vi "5_VisualAD_HyperParam_Search.vi"() -> ()   [LabVIEW 2020]
uses:
  <vilib>/Ngene/DeepLTK Anomaly Detection Addon/DeepLTK_Anomaly_Detection_Addon/API/Controls/NNPC_Coreset_Params.ctl
  <vilib>/Ngene/DeepLTK Anomaly Detection Addon/DeepLTK_Anomaly_Detection_Addon/API/Controls/NNPC_Setup.ctl
  <vilib>/Ngene/Deep Learning Toolkit/Toolkit/NN_Data/API/NN_Dims(C,H,W).ctl
  <vilib>/Ngene/Deep Learning Toolkit/Toolkit/NN_Network/Controls/NN_Device.ctl
  <vilib>/Ngene/DeepLTK Anomaly Detection Addon/DeepLTK_Anomaly_Detection_Addon/API/Controls/Feature_Scorer_Params.ctl
  <vilib>/Ngene/DeepLTK Anomaly Detection Addon/DeepLTK_Anomaly_Detection_Addon/API/Controls/Gaussian_Blur.ctl
  <vilib>/Ngene/DeepLTK Anomaly Detection Addon/DeepLTK_Anomaly_Detection_Addon/API/Controls/Evaluation_Metrics.ctl
  <vilib>/Ngene/DeepLTK Anomaly Detection Addon/DeepLTK_Anomaly_Detection_Addon/API/Controls/Eval_Results.ctl
  <vilib>/Ngene/DeepLTK Anomaly Detection Addon/DeepLTK_Anomaly_Detection_Addon/API/Controls/MinMax.ctl
  <vilib>/Ngene/DeepLTK Anomaly Detection Addon/DeepLTK_Anomaly_Detection_Addon/API/Controls/NNPC_Random_Projection_CFG.ctl
  <vilib>/Ngene/DeepLTK Anomaly Detection Addon/DeepLTK_Anomaly_Detection_Addon/API/Controls/Dim_Reduction_Method.ctl
  <vilib>/Ngene/DeepLTK Anomaly Detection Addon/DeepLTK_Anomaly_Detection_Addon/API/Controls/NNFE_CFG.ctl
  <vilib>/Ngene/DeepLTK Anomaly Detection Addon/DeepLTK_Anomaly_Detection_Addon/API/Controls/Layer_Selector.ctl
  <vilib>/Ngene/DeepLTK Anomaly Detection Addon/DeepLTK_Anomaly_Detection_Addon/API/Controls/Feature_Layer_Selector.ctl
  <vilib>/Ngene/DeepLTK Anomaly Detection Addon/DeepLTK_Anomaly_Detection_Addon/API/Controls/Interpolation_Selector.ctl
  subVIs/Dataset_Reader/Controls/Read_Options.ctl
  <vilib>/Ngene/DeepLTK Anomaly Detection Addon/DeepLTK_Anomaly_Detection_Addon/API/Controls/NNPC_PreProcessing_Options.ctl
  <vilib>/Ngene/DeepLTK Anomaly Detection Addon/DeepLTK_Anomaly_Detection_Addon/API/Controls/NNPC_DS_Stats.ctl
  <vilib>/Ngene/DeepLTK Anomaly Detection Addon/DeepLTK_Anomaly_Detection_Addon/API/Controls/Image_Stats_RGB.ctl
  subVIs/HyperParam_Investigation/Controls/Model_Info_and_Report.ctl
  subVIs/HyperParam_Investigation/Controls/Feature_Layers_CFG.ctl
  <vilib>/Ngene/DeepLTK Anomaly Detection Addon/DeepLTK_Anomaly_Detection_Addon/API/Controls/Eval_Config.ctl
  <vilib>/Ngene/DeepLTK Anomaly Detection Addon/DeepLTK_Anomaly_Detection_Addon/API/NNPC_Generate_Embedding/NNPC_Generate_Embedding(Dataset).vi
  <vilib>/Ngene/DeepLTK Anomaly Detection Addon/DeepLTK_Anomaly_Detection_Addon/API/NNPC_Predict/NNPC_Predict(Dataset).vi
  <vilib>/Ngene/Deep Learning Toolkit/Toolkit/NN_Data/subVIs/Dataset_Destroy/NN_Dataset_Destroy(In3D_Out3D).vi
  <vilib>/Ngene/DeepLTK Anomaly Detection Addon/DeepLTK_Anomaly_Detection_Addon/API/Controls/NNPC_Save_CFG.ctl
  <vilib>/Ngene/DeepLTK Anomaly Detection Addon/DeepLTK_Anomaly_Detection_Addon/DeepLTK_Anomaly_Detection_Addon.lvlib
  <vilib>/Ngene/Deep Learning Toolkit/Toolkit/Deep_Learning_Toolkit_by_Ngene.lvlib
panel:
  in  "Tab Control":enum32{"Setup", "Results"}(tab)=enum."Results"
  in  "Min_Layers_In_Group":u16=2
  in  "Dataset_Path(Train/Test/GT)":path=path "D:/DNN/_from_Customer/2025_04_11_NIConnect_PCB5/1_Dataset/20_10_Train_2BG_Append_2025_04_21"
  in  "PatchCore_Dest_Folder_Path":path=path "D:/working/HPO_PCB5_Large/RN18"
  in  "Coreset_Size":sgl[](array[numeric])=[15000.0, 20000.0, 25000.0]
  in  "Image Res.":i32[](array[numeric])=[448, 464, 480]
  in  "Proj._Dim.":i32[](array[numeric])=[300]
  in  "Coreset_Params":T1={"CoreSet_Size"=2000.0, "Start_idx"=3}
  in  "NNPC_Setup":T2={"Input_Dims"={"C"=3, "H"=224, "W"=224}, "mBatch"=1, "Device"=enum."GPU", "GPU Id"=0}
  in  "Feature_Scorer_Params":T5={"Nearest_Neighbors"=1, "Calculate Anomaly Map"=FALSE, "Gaussian_Blur"={"Kernel_Size"=33, "Sigma"=4.0}}
  in  "Dim Reduction":T7={"Method"=enum."Rnd_Proj", "Target_Dim"=-1, "Seed"=42}
  in  "NNFE_CFG":T9={"Name"="AD_PCB4", "Layer_Selection_By"=enum."Stride", "Feature_Layers"={"[LayerID, PatchSize]"=[{"Layer_ID"=8, "Patch_Size"=3}, {"Layer_ID"=16, "Patch_Size"=3}]}, "Interpolation_Type"=enum."Bi-Linear"}
  in  "NNFE_Folder_Paths":path[](array[path])=[path "D:/Ngene/Projects_SVN/AD/Models/0_Orig/RN18_1", path "D:/Ngene/Projects_SVN/AD/Models/0_Orig/RN18_2", path "D:/Ngene/Projects_SVN/AD/Models/0_Orig/RN18_3"]
  in  "Patch Sizes":i32[](array[numeric])=[1, 3, 5]
  in  "Layer IDs":i32[](array[numeric])=[8, 16]
  out "Feature_Layers":T11[](array[typedef])=[{"[LayerID, PatchSize]"=[{"Layer_ID"=16, "Patch_Size"=1}]}, {"[LayerID, PatchSize]"=[{"Layer_ID"=16, "Patch_Size"=3}]}, {"[LayerID, PatchSize]"=[{"Layer_ID"=16, "Patch_Size"=5}]}, {"[LayerID, PatchSize]"=[{"Layer_ID"=8, "Patch_Size"=1}]}, {"[LayerID, PatchSize]"=[{"Layer_ID"=8, "Patch_Size"=1}, {"Layer_ID"=16, "Patch_Size"=1}]}, {"[LayerID, PatchSize]"=[{"Layer_ID"=8, "Patch_Size"=1}, {"Layer_ID"=16, "Patch_Size"=3}]}, {"[LayerID, PatchSize]"=[{"Layer_ID"=8, "Patch_Size"=1}, {"Layer_ID"=16, "Patch_Size"=5}]}, {"[LayerID, PatchSize]"=[{"Layer_ID"=8, "Patch_Size"=3}]}, {"[LayerID, PatchSize]"=[{"Layer_ID"=8, "Patch_Size"=3}, {"Layer_ID"=16, "Patch_Size"=1}]}, {"[LayerID, PatchSize]"=[{"Layer_ID"=8, "Patch_Size"=3}, {"Layer_ID"=16, "Patch_Size"=3}]}, {"[LayerID, PatchSize]"=[{"Layer_ID"=8, "Patch_Size"=3}, {"Layer_ID"=16, "Patch_Size"=5}]}, {"[LayerID, PatchSize]"=[{"Layer_ID"=8, "Patch_Size"=5}]}, {"[LayerID, PatchSize]"=[{"Layer_ID"=8, "Patch_Size"=5}, {"Layer_ID"=16, "Patch_Size"=1}]}, {"[LayerID, PatchSize]"=[{"Layer_ID"=8, "Patch_Size"=5}, {"Layer_ID"=16, "Patch_Size"=3}]}, {"[LayerID, PatchSize]"=[{"Layer_ID"=8, "Patch_Size"=5}, {"Layer_ID"=16, "Patch_Size"=5}]}]
  in  "Max_Layers_In_Group":u16=2
  out "Max_Dist":sgl[](graph)
  out "Total Iters":i32=135
  out "Current Iter":i32=1
  out "Coreset Size":i32=3
  out "Proj. Dim.":i32=1
  out "Img Res.":i32=3
  out "Feature_Layers":i32=15
  out "Elapsed Time":dbl=86.03153250000014 format="%<%H:%M:%S>t"
  out "Evaluation_Metrics(Image)":T13={"Scores(Good)"={"X Values"=[2.7319342923164367, 2.7571603751182554, 2.7823864579200746, 2.8076125407218933, 2.8328386235237124, 2.858064706325531, 2.88329078912735, 2.9085168719291685, 2.9337429547309877, 2.9589690375328064, 2.9841951203346255, 3.0094212031364442, 3.034647285938263, 3.0598733687400816, 3.0850994515419004, 3.1103255343437195, 3.1355516171455386, 3.1607776999473574, 3.186003782749176, 3.2112298655509948, 3.2364559483528135, 3.2616820311546326, 3.2869081139564513, 3.3121341967582705, 3.337360279560089, 3.362586362361908, 3.3878124451637266, 3.4130385279655457, 3.4382646107673644, 3.4634906935691836, 3.4887167763710023, 3.513942859172821, 3.5391689419746397, 3.5643950247764584, 3.5896211075782776, 3.6148471903800967, 3.6400732731819154, 3.665299355983734, 3.690525438785553, 3.7157515215873715, 3.7409776043891907, 3.76620368719101, 3.7914297699928285, 3.8166558527946473, 3.841881935596466, 3.8671080183982847, 3.8923341012001034, 3.917560184001923, 3.9427862668037417, 3.9680123496055604, 3.993238432407379, 4.018464515209198, 4.0436905980110165, 4.068916680812835, 4.094142763614655, 4.1193688464164735, 4.144594929218292, 4.169821012020111, 4.1950470948219305, 4.220273177623749, 4.245499260425568, 4.270725343227387, 4.295951426029205, 4.321177508831024, 4.346403591632843, 4.371629674434661, 4.39685575723648, 4.4220818400383, 4.447307922840118, 4.472534005641937, 4.497760088443756, 4.5229861712455754, 4.548212254047394, 4.573438336849213, 4.598664419651032, 4.62389050245285, 4.649116585254669, 4.674342668056488, 4.699568750858306, 4.724794833660126, 4.750020916461945, 4.775246999263763, 4.800473082065583, 4.825699164867402, 4.85092524766922, 4.876151330471039, 4.901377413272858, 4.9266034960746765, 4.951829578876495, 4.977055661678314, 5.002281744480133, 5.027507827281951, 5.05273391008377, 5.07795999288559, 5.103186075687408, 5.128412158489228, 5.153638241291047, 5.178864324092865, 5.204090406894684, 5.229316489696503], "Histogram: h(x)"=[1, 0, 0, 0, 1, 1, 0, 0, 0, 0, 0, 2, 2, 2, 5, 9, 13, 20, 27, 26, 18, 22, 13, 22, 8, 15, 14, 13, 5, 4, 7, 3, 5, 1, 2, 0, 4, 3, 1, 1, 3, 1, 0, 0, 1, 0, 1, 3, 0, 3, 2, 1, 1, 2, 0, 0, 0, 1, 0, 1, 0, 1, 0, 0, 0, 1, 0, 0, 0, 0, 0, 0, 0, 0, 1, 0, 0, 1, 0, 0, 0, 0, 0, 0, 0, 0, 0, 0, 0, 0, 1, 0, 0, 0, 1, 0, 1, 0, 0, 0]}, "Scores(Bad)"={"X Values"=[2.7319342923164367, 2.7571603751182554, 2.7823864579200746, 2.8076125407218933, 2.8328386235237124, 2.858064706325531, 2.88329078912735, 2.9085168719291685, 2.9337429547309877, 2.9589690375328064, 2.9841951203346255, 3.0094212031364442, 3.034647285938263, 3.0598733687400816, 3.0850994515419004, 3.1103255343437195, 3.1355516171455386, 3.1607776999473574, 3.186003782749176, 3.2112298655509948, 3.2364559483528135, 3.2616820311546326, 3.2869081139564513, 3.3121341967582705, 3.337360279560089, 3.362586362361908, 3.3878124451637266, 3.4130385279655457, 3.4382646107673644, 3.4634906935691836, 3.4887167763710023, 3.513942859172821, 3.5391689419746397, 3.5643950247764584, 3.5896211075782776, 3.6148471903800967, 3.6400732731819154, 3.665299355983734, 3.690525438785553, 3.7157515215873715, 3.7409776043891907, 3.76620368719101, 3.7914297699928285, 3.8166558527946473, 3.841881935596466, 3.8671080183982847, 3.8923341012001034, 3.917560184001923, 3.9427862668037417, 3.9680123496055604, 3.993238432407379, 4.018464515209198, 4.0436905980110165, 4.068916680812835, 4.094142763614655, 4.1193688464164735, 4.144594929218292, 4.169821012020111, 4.1950470948219305, 4.220273177623749, 4.245499260425568, 4.270725343227387, 4.295951426029205, 4.321177508831024, 4.346403591632843, 4.371629674434661, 4.39685575723648, 4.4220818400383, 4.447307922840118, 4.472534005641937, 4.497760088443756, 4.5229861712455754, 4.548212254047394, 4.573438336849213, 4.598664419651032, 4.62389050245285, 4.649116585254669, 4.674342668056488, 4.699568750858306, 4.724794833660126, 4.750020916461945, 4.775246999263763, 4.800473082065583, 4.825699164867402, 4.85092524766922, 4.876151330471039, 4.901377413272858, 4.9266034960746765, 4.951829578876495, 4.977055661678314, 5.002281744480133, 5.027507827281951, 5.05273391008377, 5.07795999288559, 5.103186075687408, 5.128412158489228, 5.153638241291047, 5.178864324092865, 5.204090406894684, 5.229316489696503], "Histogram: h(x)"=[0, 0, 0, 0, 0, 0, 0, 0, 0, 0, 0, 0, 0, 0, 0, 0, 0, 0, 0, 0, 0, 0, 0, 0, 0, 0, 0, 0, 1, 0, 1, 0, 2, 1, 3, 1, 2, 6, 5, 4, 2, 0, 6, 6, 8, 6, 6, 8, 5, 7, 6, 6, 4, 6, 4, 6, 6, 8, 7, 2, 4, 6, 4, 5, 2, 3, 7, 1, 6, 1, 1, 1, 1, 1, 4, 1, 3, 5, 1, 0, 1, 1, 2, 1, 1, 1, 0, 0, 0, 0, 0, 0, 0, 0, 0, 0, 0, 0, 0, 1]}, "Eval Stats"={"Scores(Good)"={"Min"=2.7193213, "Max"=5.1506834}, "Scores(Bad)"={"Min"=3.4291687, "Max"=5.2419295}, "# of Samples(Good)"=297, "# of Samples(Bad)"=200, "AUROC"=0.95147306, "F1_Max"=0.90410954, "Thrshld(F1_Max)"=3.54504, "Prec.(F1_Max)"=0.8319328, "Recall(F1_Max)"=0.99, "FPR(F1_Max)"=0.13468014, "FNR(F1_Max)"=0.01}} {"Eval Stats"."Recall(F1_Max)" format="%#.5f"; "Eval Stats"."FPR(F1_Max)" format="%#.5f"; "Eval Stats"."FNR(F1_Max)" format="%#.5f"; "Eval Stats"."Prec.(F1_Max)" format="%#.5f"; "Eval Stats"."F1_Max" format="%#.5f"; "Eval Stats"."AUROC" format="%#.5f"; "Eval Stats"."Scores(Bad)"."Min" format="%#_5g"; "Eval Stats"."Scores(Good)"."Min" format="%#_5g"; "Eval Stats"."Thrshld(F1_Max)" format="%#_5f"}
  out "Evaluation_Metrics(Pixel)":T13 {"Eval Stats"."Recall(F1_Max)" format="%#.5f"; "Eval Stats"."FPR(F1_Max)" format="%#.5f"; "Eval Stats"."FNR(F1_Max)" format="%#.5f"; "Eval Stats"."Prec.(F1_Max)" format="%#.5f"; "Eval Stats"."F1_Max" format="%#.5f"; "Eval Stats"."AUROC" format="%#.5f"; "Eval Stats"."Scores(Bad)"."Min" format="%#_5g"; "Eval Stats"."Scores(Good)"."Min" format="%#_5g"; "Eval Stats"."Thrshld(F1_Max)" format="%#_5f"}
  out "Coreset Size":i32=1
  out "Coreset Size":sgl=20000.0
  out "Proj. Dim.":i32=300
  out "Img. Res.":i32=448
  out "Proj. Dim.":i32
  out "Img Res.":i32
  out "dT_Eval":dbl=0.21638530000018363 format="%#_4p"
  out "dT_Inference":dbl=0.004835436016095979 format="%#_4p"
  out "dT_Coreset":dbl=52.57081759999983 format="%#_4p"
  out "dT_Embed":dbl=4.344940299999962 format="%#_3p"
  out "dT_Init":dbl=0.7978293999999551 format="%#_3p"
  out "dT_DS_Read(Test)":dbl=6.224915199999941 format="%#_3p"
  out "dT_DS_Read(Train)":dbl=16.388801800000238 format="%#_3p"
  out "DS Size(Test)":i32=497
  out "DS Size(Train)":i32=1036
  out "Feature_Layers":i32
  out "error out":errorcluster
  out "dT_DS_Read(Train)":dbl=48.993010699999985
  out "dT_DS_Read(Test)":dbl=18.836170100000004
  out "dT_Init":dbl=2.419111600000008
  out "dT_Predict":dbl=8.196476700000034
  out "dT_Coreset":dbl=154.10587869999995
  out "dT_Embed":dbl=13.308446900000035
  out "dT_Eval":dbl=0.7761126999999419
  out "Feature Extractor":string="rn18_2"
  out "dT_Predict":dbl=2.4032116999997015
  out "[LayerID, PatchSize]":cluster{"Layer_ID":i32, "Patch_Size":i32}[](array[cluster])=[{"Layer_ID"=16, "Patch_Size"=1}]
  in  "Stop":bool
  out "NNFE":i32=1
  out "NNFE":i32=3
  # "Total Iterations"
  # "Current Iteration"
  # "Current Settings"
  # "Total Times"
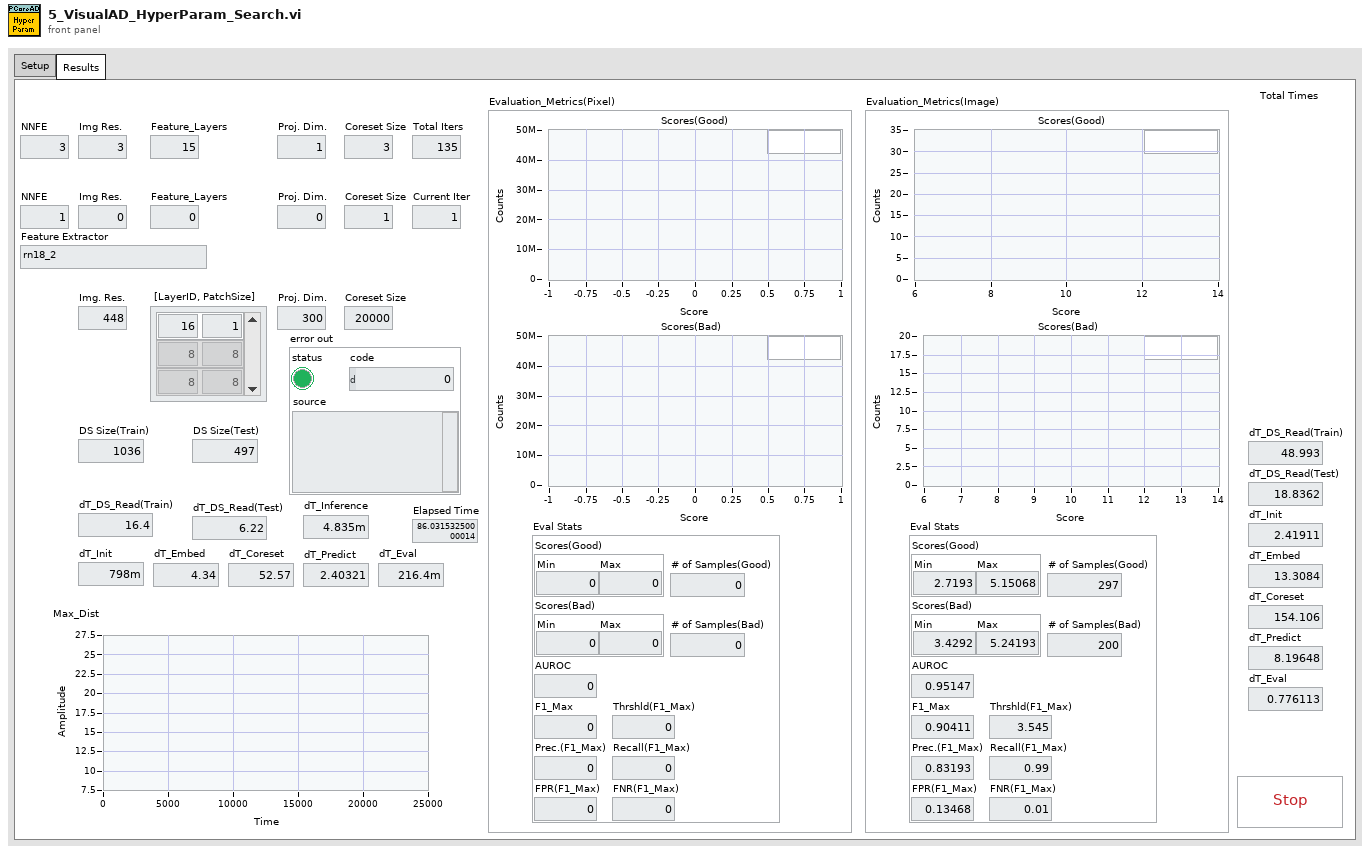
[diagram p1: front panel]
types:
  T1 = typedef "DeepLTK_Anomaly_Detection_Addon.lvlib/NNPC_Coreset_Params.ctl" = cluster{"CoreSet_Size":sgl, "Start_idx":i32}
  T2 = typedef "DeepLTK_Anomaly_Detection_Addon.lvlib/NNPC_Setup.ctl" = cluster{"Input_Dims":T3, "mBatch":i32, "Device":T4, "GPU Id":i32}
  T3 = typedef "Deep_Learning_Toolkit_by_Ngene.lvlib/NN_Dims(C,H,W).ctl" = cluster{"C":i32, "H":i32, "W":i32}
  T4 = typedef "Deep_Learning_Toolkit_by_Ngene.lvlib/NN_Device.ctl" = enum16{"CPU", "GPU"}
  T5 = typedef "DeepLTK_Anomaly_Detection_Addon.lvlib/Feature_Scorer_Params.ctl" = cluster{"Nearest_Neighbors":i32, "Calculate Anomaly Map":bool, "Gaussian_Blur":T6}
  T6 = typedef "DeepLTK_Anomaly_Detection_Addon.lvlib/Gaussian_Blur.ctl" = cluster{"Kernel_Size":i32, "Sigma":sgl}
  T7 = typedef "DeepLTK_Anomaly_Detection_Addon.lvlib/NNPC_Random_Projection_CFG.ctl" = cluster{"Method":T8, "Target_Dim":i32, "Seed":i32}
  T8 = typedef "DeepLTK_Anomaly_Detection_Addon.lvlib/Dim_Reduction_Method.ctl" = enum16{"None", "Rnd_Proj", "PCA"}
  T9 = typedef "DeepLTK_Anomaly_Detection_Addon.lvlib/NNFE_CFG.ctl" = cluster{"Name":string, "Layer_Selection_By":T10, "Feature_Layers":T11, "Interpolation_Type":T12}
  T10 = typedef "DeepLTK_Anomaly_Detection_Addon.lvlib/Layer_Selector.ctl" = enum16{"Stride", "Layer_Idx"}
  T11 = typedef "DeepLTK_Anomaly_Detection_Addon.lvlib/Feature_Layer_Selector.ctl" = cluster{"[LayerID, PatchSize]":cluster{"Layer_ID":i32, "Patch_Size":i32}[]}
  T12 = typedef "DeepLTK_Anomaly_Detection_Addon.lvlib/Interpolation_Selector.ctl" = enum16{"Nearest", "Bi-Linear"}
  T13 = typedef "DeepLTK_Anomaly_Detection_Addon.lvlib/Evaluation_Metrics.ctl" = cluster{"Scores(Good)":cluster{"X Values":dbl[], "Histogram: h(x)":i32[]}, "Scores(Bad)":cluster{"X Values":dbl[], "Histogram: h(x)":i32[]}, "Eval Stats":T14}
  T14 = typedef "DeepLTK_Anomaly_Detection_Addon.lvlib/Eval_Results.ctl" = cluster{"Scores(Good)":T15, "Scores(Bad)":T15, "# of Samples(Good)":i32, "# of Samples(Bad)":i32, "AUROC":sgl, "F1_Max":sgl, "Thrshld(F1_Max)":sgl, "Prec.(F1_Max)":sgl, "Recall(F1_Max)":sgl, "FPR(F1_Max)":sgl, "FNR(F1_Max)":sgl}
  T15 = typedef "DeepLTK_Anomaly_Detection_Addon.lvlib/MinMax.ctl" = cluster{"Min":sgl, "Max":sgl}
  T16 = typedef "DeepLTK_Anomaly_Detection_Addon.lvlib/NN_Paths.ctl" = cluster{"CFG":path, "BIN":path}
  T17 = typedef "DeepLTK_Anomaly_Detection_Addon.lvlib/NNPC_PreProcessing_Options.ctl" = cluster{"DS_Name":string, "Input_Dims":T3, "Center Crop Size":i32, "Interpolation Type":u32, "Multi-Stage_DownSample?":bool, "Dataset_Stats":T18}
  T18 = typedef "DeepLTK_Anomaly_Detection_Addon.lvlib/NNPC_DS_Stats.ctl" = cluster{"means":T19, "stds":T19}
  T19 = typedef "DeepLTK_Anomaly_Detection_Addon.lvlib/Image_Stats_RGB.ctl" = cluster{"R":sgl, "G":sgl, "B":sgl}
  T20 = typedef "Read_Options.ctl" = cluster{"Read Bads?":bool, "Read GTs?":bool, "Update. DS Stats?":bool}
  T21 = typedef "DeepLTK_Anomaly_Detection_Addon.lvlib/Eval_Config.ctl" = cluster{"Extract_Good_Pixels_from_Bad":bool, "# bins":i32}
  T22 = typedef "Model_Info_and_Report.ctl" = cluster{"Name":string, "Feature Extractor":string, "Input3D_Custom_Dims":T3, "Coreset Size":i32, "J-L Proj. Dim.":i32, "Train_Time":dbl, "Inf_Time":dbl, "Feature_Layers":T23, "Eval Stats(Image)":T14, "Eval Stats(Pixel)":T14}
  T23 = typedef "Feature_Layers_CFG.ctl" = cluster{"Layer_ID":i32, "Patch_Size":i32}[]
  T24 = typedef "DeepLTK_Anomaly_Detection_Addon.lvlib/NNPC_Save_CFG.ctl" = cluster{"Add_TimeStamp_SubFolder":bool, "Append_TimeStamp_to_FileNames":bool}
  T25 = typedef "Deep_Learning_Toolkit_by_Ngene.lvlib/NN_DataSet(In3D_Out3D).ctl" = cluster{"Dataset_Size":i32, "Dims_In":T3, "Labels":string[], "File Paths":path[], "Outputs Ref.":T26, "Inputs Ref.":variant, "Dims_Out":T3}
  T26 = typedef "Deep_Learning_Toolkit_by_Ngene.lvlib/NN_Data_ref(4D_SGL).ctl" = refnum<data-value>
  T27 = typedef "DeepLTK_Anomaly_Detection_Addon.lvlib/NNPC_Instance.ctl" = cluster{"NN":T28, "MemBank_Data":T43, "Name":string}
  T28 = typedef "Deep_Learning_Toolkit_by_Ngene.lvlib/NN.ctl" = cluster{"Name":string, "No of Layers":i32, "mBatch":i32, "Layers":T29[], "Dimty":T30, "Dims_In":T3, "Dims_Out":T3, "Working_Dir":path, "Train?":bool, "Train_Params":T31, "LR_Update_Policy":T34, "Session Data":T36, "Ground_truth":T37, "NNg_hdls":T38, "NN_Device":T4, "GPU Id":i32, "Labels":string[], "Receptive Field":T39[], "Loss_Type":T40, "Loss_Cfg_Prms":variant, "NNG_WS":T41}
  T29 = typedef "Deep_Learning_Toolkit_by_Ngene.lvlib/NN_Layer_ref.ctl" = refnum<data-value>
  T30 = typedef "Deep_Learning_Toolkit_by_Ngene.lvlib/NN_In_Out_Dim-ty.ctl" = enum8{"In1D_Out1D", "In3D_Out1D", "In3D_Out3D", "In3D_OutBBox"}
  T31 = typedef "Deep_Learning_Toolkit_by_Ngene.lvlib/NN_Train_Params.ctl" = cluster{"Optimizer":T32, "Beta_1":sgl, "Beta_2":sgl, "Weight Decay(L1)":sgl, "Weight Decay(L2)":sgl, "Data_Sampling":T33}
  T32 = typedef "Deep_Learning_Toolkit_by_Ngene.lvlib/NN_Train_Optimizer.ctl" = enum16{"SGD", "Adam", "Adagrad", "Adadelta", "RMSProp", "Nesterov"}
  T33 = typedef "Deep_Learning_Toolkit_by_Ngene.lvlib/NN_Train_Data_Sampling.ctl" = enum16{"Random", "Sequential"}
  T34 = typedef "Deep_Learning_Toolkit_by_Ngene.lvlib/NN_LR_Policy_Cfg.ctl" = cluster{"Policy_Type":T35, "LR0":dbl, "k":sgl, "WarmUp_Policy":enum16{"Step", "Ramp"}, "WarmUp_Iter":i32, "WarmUp_Ratio":sgl}
  T35 = typedef "Deep_Learning_Toolkit_by_Ngene.lvlib/NN_LR_Policy_Type.ctl" = enum16{"Manual", "Step", "Exp", "1/t"}
  T36 = typedef "Deep_Learning_Toolkit_by_Ngene.lvlib/NN_Train_Session_Data.ctl" = cluster{"Epochs":sgl, "Tot_Iter":i32, "LR":sgl, "LR_iter":i32}
  T37 = typedef "Deep_Learning_Toolkit_by_Ngene.lvlib/NN_Ground_truth.ctl" = cluster{"Y":variant}
  T38 = typedef "Deep_Learning_Toolkit_by_Ngene.lvlib/nng_cuda_handles.ctl" = cluster{"cudnn":u64, "cublas":u64, "stream":u64, "curand":u64}
  T39 = typedef "Deep_Learning_Toolkit_by_Ngene.lvlib/NN_Dims(V,H).ctl" = cluster{"V":i32, "H":i32}
  T40 = typedef "Deep_Learning_Toolkit_by_Ngene.lvlib/NN_Loss_Type.ctl" = enum16{"None", "MSE", "CrossEntropy", "YOLO_v2", "YOLO_v4"}
  T41 = typedef "Deep_Learning_Toolkit_by_Ngene.lvlib/NNG_WS.ctl" = cluster{"NNG_WS_Mem":T42, "Max_WS_Size":i64}
  T42 = typedef "Deep_Learning_Toolkit_by_Ngene.lvlib/NNg_WS_Mem_DVR.ctl" = refnum<data-value>
  T43 = typedef "DeepLTK_Anomaly_Detection_Addon.lvlib/MemBank_and_Norm_Variants.ctl" = cluster{"MemBank":variant, "MemBank Norm":variant}
  T44 = typedef "DeepLTK_Anomaly_Detection_Addon.lvlib/Evaluation_Metrics(Pixel_Image).ctl" = cluster{"Evaluation_Metrics(Pixel)":T13, "Evaluation_Metrics(Image)":T13}
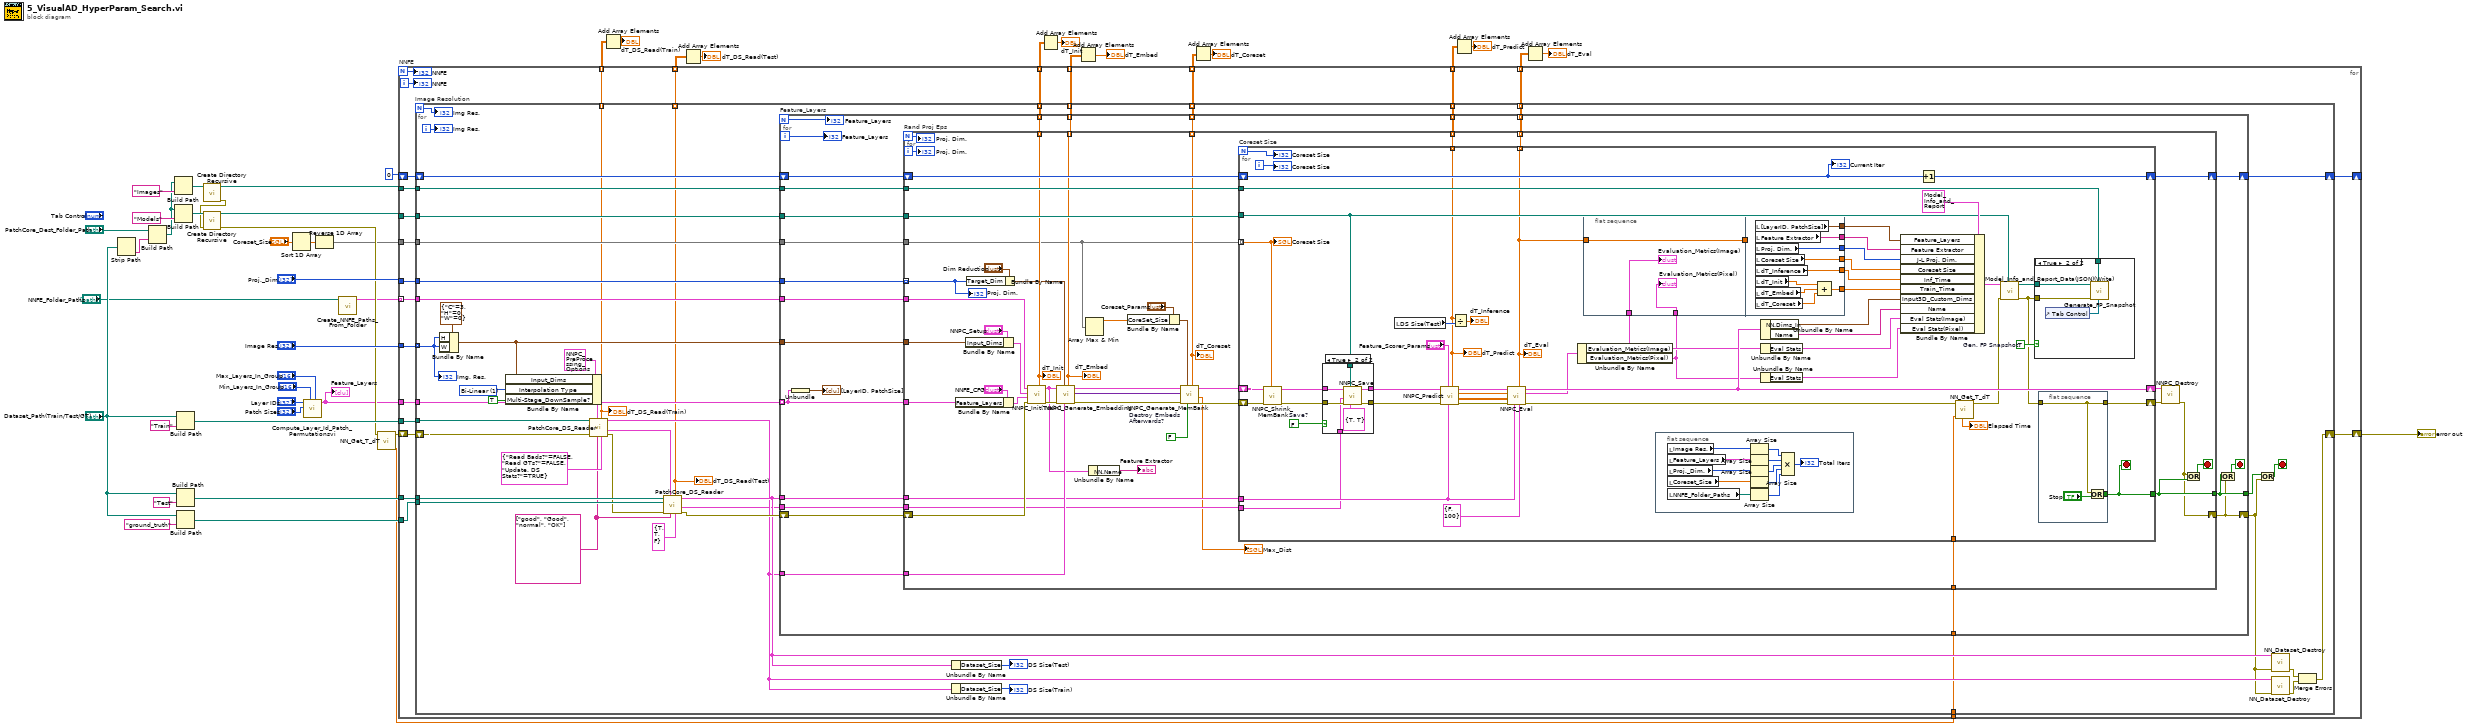
[diagram p0: block diagram]
diagram:
  n1 = Strip Path(path="Dataset_Path(Train/Test/GT)") -> (name=w43:string)  [unwired: 1 out]
  n2 = Build Path(base path="PatchCore_Dest_Folder_Path", name or relative path=w43) -> (appended path=w33:path)
  n3 = Build Path(base path=w33, name or relative path="Images" ("String")) -> (appended path=w37:path)
  n4 = Build Path(base path=w33, name or relative path="Models" ("String")) -> (appended path=w36:path)
  n5 = Build Path(base path="Dataset_Path(Train/Test/GT)", name or relative path="Train" ("String")) -> (appended path=w38:path)
  n6 = Build Path(base path="Dataset_Path(Train/Test/GT)", name or relative path="Test" ("String")) -> (appended path=w39:path)
  n7 = Build Path(base path="Dataset_Path(Train/Test/GT)", name or relative path="ground_truth" ("String")) -> (appended path=w44:path)
  n8 = call <vilib>:"Create Directory Recursive.vi"("directory"=w37) -> ("error out"=w29:errorcluster, "directory copy"=w31:path)  [unwired: 4 in, 1 out]
  n9 = call <vilib>:"Create Directory Recursive.vi"("error in (no error)"=w29, "directory"=w36) -> ("error out"=w28:errorcluster, "directory copy"=w32:path)  [unwired: 3 in, 1 out]
  n10 = Sort 1D Array(array="Coreset_Size") -> (sorted array=w15:sgl[])
  n11 = call "Compute_Layer_Id_Patch_Permutationsvi.vi"("Max Layers"="Max_Layers_In_Group", "Min Layers"="Min_Layers_In_Group", "Patch Sizes"="Patch Sizes", "Layer IDs"="Layer IDs") -> ("LayerID,PatchSize Permutations"=w3:T11[])  [unwired: 7 in]
  "Feature_Layers" <- w3
  n12 = Reverse 1D Array(array=w15) -> (reversed array=w14:sgl[])
  n13 = call "Create_NNFE_Paths_From_Folder.vi"("NNFE_Folder_Paths"="NNFE_Folder_Paths") -> ("NNFE_File_Paths"=w10:T16[])  [unwired: 10 in]
  n14 = call <vilib>:"NN_Get_T_dT.vi"("error in (no error)"=w28) -> ("T_out"=w30:dbl, "error out"=w11:errorcluster)  [unwired: 6 in, 1 out]
  n15 = for "NNFE" {
    N -> [w50]
    tunnel: "Image Res." -> [w72]
    tunnel: w44 -> [w71]
    tunnel: "Proj._Dim." -> [w70]
    tunnel: w39 -> [w69]
    tunnel: w38 -> [w68]
    tunnel: w32 -> [w67]
    tunnel: w31 -> [w66]
    tunnel: w30 -> [w65]
    tunnel: w3 -> [w64]
    tunnel: [w62] -> w26 mode=indexing
    tunnel: [w61] -> w25 mode=indexing
    tunnel: [w60] -> w24 mode=indexing
    tunnel: [w59] -> w23 mode=indexing
    tunnel: [w58] -> w22 mode=indexing
    tunnel: w14 -> [w57]
    shift-right: [w56] -> w12
    shift-left: w11 -> [w55]
    tunnel: w10 -> [w54] mode=indexing
    shift-right: [w53] -> _
    shift-left: 0 ("Img. Res. 2") -> [w63]
    tunnel: [w52] -> w8 mode=indexing
    tunnel: [w51] -> w6 mode=indexing
    i -> [w49]
    n16 = for "Image Resolution" {
      N -> [w90]
      tunnel: w71 -> [w112]
      tunnel: w68 -> [w113]
      tunnel: w72 -> [w115] mode=indexing
      tunnel: w70 -> [w117]
      tunnel: w57 -> [w116]
      tunnel: w69 -> [w111]
      shift-right: [w99] -> w56
      shift-left: w55 -> [w114]
      tunnel: w67 -> [w102]
      tunnel: w66 -> [w101]
      tunnel: w65 -> [w100]
      tunnel: w64 -> [w91]
      shift-right: [w87] -> w53
      shift-left: w63 -> [w88]
      tunnel: [w75] -> w62 mode=indexing
      tunnel: [w74] -> w61 mode=indexing
      tunnel: [w86] -> w60 mode=indexing
      tunnel: [w85] -> w52 mode=indexing
      tunnel: [w84] -> w59 mode=indexing
      tunnel: [w83] -> w58 mode=indexing
      tunnel: [w82] -> w51 mode=indexing
      tunnel: w54 -> [w76]
      i -> [w118]
      stop <- w81 stop-if-true
      w97 = u32 1 items=["Zero Order", "Bi-Linear", "Quadratic", "Cubic Spline"] ("Interpolation Type")
      w77 = string[] ["good", "Good", "normal", "OK"] ("Good Folder Name")
      n17 = Bundle By Name(cluster=T3 {"C"=3, "H"=0, "W"=0} ("Input_Dims"), "H"=w115, "W"=w115) -> (w92:T3)
      n18 = Bundle By Name(cluster=T17 {"DS_Name"="", "Input_Dims"={"C"=4, "H"=224, "W"=224}, "Center Crop Size"=-1, "Interpolation Type"=1, "Multi-Stage_DownSample?"=FALSE, "Dataset_Stats"={"means"={"R"=0.5385, "G"=0.5348, "B"=0.551}, "stds"={"R"=0.3673, "G"=0.3673, "B"=0.3505}}} ("PreProcessing_Options"), "Input_Dims"=w92, "Interpolation Type"=w97, "Multi-Stage_DownSample?"=TRUE) -> (w79:T17)
      n19 = call "PatchCore_DS_Reader.vi"("Read Options"=T20 {"Read Bads?"=FALSE, "Read GTs?"=FALSE, "Update. DS Stats?"=TRUE}, "Good Unique Labels"=w77, "PreProc_Options_in"=w79, "error in (no error)"=w114, "Folder Path"=w113) -> ("error out"=w110:errorcluster, "PreProc_Options_out"=w78:T17, "Dataset"=w104:T25, "dT_DS_Reader"=w75:dbl)  [unwired: 3 in]
      "dT_DS_Read(Train)" <- w75
      n20 = call "PatchCore_DS_Reader.vi"("Read Options"=T20 {"Read Bads?"=TRUE, "Read GTs?"=TRUE, "Update. DS Stats?"=FALSE}, "Good Unique Labels"=w77, "PreProc_Options_in"=w78, "error in (no error)"=w110, "GT Folder Path"=w112, "Folder Path"=w111) -> ("error out"=w108:errorcluster, "PreProc_Options_out"=w94:T17, "Dataset"=w105:T25, "dT_DS_Reader"=w74:dbl)  [unwired: 2 in]
      "dT_DS_Read(Test)" <- w74
      n21 = for "Feature_Layers" {
        N -> [w131]
        tunnel: w117 -> [w143]
        tunnel: w116 -> [w142]
        tunnel: w105 -> [w140]
        tunnel: w104 -> [w139]
        tunnel: w102 -> [w138]
        tunnel: w101 -> [w137]
        tunnel: w100 -> [w136]
        tunnel: w94 -> [w135]
        shift-right: [w121] -> w80
        shift-left: w108 -> [w141]
        tunnel: w92 -> [w133]
        tunnel: w91 -> [w132] mode=indexing
        tunnel: [w130] -> w89
        shift-right: [w129] -> w87
        shift-left: w88 -> [w128]
        tunnel: [w127] -> w86 mode=indexing
        tunnel: [w126] -> w85 mode=indexing
        tunnel: [w125] -> w84 mode=indexing
        tunnel: [w124] -> w83 mode=indexing
        tunnel: [w123] -> w82 mode=indexing
        tunnel: w76 -> [w119]
        i -> [w134]
        stop <- w122 stop-if-true
        n22 = Unbundle(w132) -> ("[LayerID, PatchSize]"=→"[LayerID, PatchSize]":cluster{"Layer_ID":i32, "Patch_Size":i32}[])
        n23 = for "Rand Proj Eps" {
          N -> [w171]
          tunnel: w138 -> [w188]
          tunnel: w139 -> [w183]
          tunnel: w143 -> [w178] mode=indexing
          tunnel: w142 -> [w146]
          shift-right: [w162] -> w121
          shift-left: w141 -> [w187]
          tunnel: w140 -> [w181]
          tunnel: w137 -> [w180]
          tunnel: w136 -> [w179]
          tunnel: w135 -> [w177]
          tunnel: w133 -> [w173]
          tunnel: w132 -> [w172]
          tunnel: [w170] -> w130
          shift-right: [w168] -> w129
          shift-left: w128 -> [w169]
          tunnel: [w167] -> w127 mode=indexing
          tunnel: [w166] -> w126 mode=indexing
          tunnel: [w150] -> w125 mode=indexing
          tunnel: [w165] -> w124 mode=indexing
          tunnel: [w164] -> w123 mode=indexing
          tunnel: w119 -> [w145]
          i -> [w186]
          stop <- w163 stop-if-true
          w154 = FALSE  # Destroy Embeds Afterwards?
          n24 = Bundle By Name(cluster="NNFE_CFG", "Feature_Layers"=w172) -> (w161:T9)
          n25 = Bundle By Name(cluster="NNPC_Setup", "Input_Dims"=w173) -> (w160:T2)
          n26 = Bundle By Name(cluster="Dim Reduction", "Target_Dim"=w178) -> (w159:T7)
          n27 = call <vilib>:"NNPC_Init(Train).vi"("error in"=w187, "NNFE_CFG"=w161, "NNPC_Setup"=w160, "NNFE_Paths"=w145) -> ("error out"=w184:errorcluster, "NNPC_out"=w158:T27, "dT_Init_Train"=w167:dbl)  [unwired: 5 in]
          "dT_Init" <- w167
          n28 = call-poly <vilib>:"NNPC_Generate_Embedding.vi"("Dataset"=w183, "Dim_Reduction"=w159, "error in"=w184, "NNPC_in"=w158) -> ("error out"=w153:errorcluster, "Feature_Embeddings"=w152:variant, "NNPC_out"=w151:T27, "dT_Embed"=w166:dbl)  [unwired: 3 in, 1 out]
          "dT_Embed" <- w166
          n29 = Array Max & Min(array=w146) -> (max value=w149:sgl)  [unwired: 3 out]
          n30 = Unbundle By Name(w158) -> ("NN.Name"=→"Feature Extractor":string)
          n31 = Bundle By Name(cluster="Coreset_Params", "CoreSet_Size"=w149) -> (w156:T1)
          n32 = call <vilib>:"NNPC_Generate_MemBank.vi"("Destroy Embeds Afterwards?"=w154, "Coreset_Params"=w156, "error in (no error)"=w153, "Feature_Embeddings"=w152, "NNPC_in"=w151) -> ("error out"=w148:errorcluster, "Max_Distances"=→"Max_Dist":sgl[], "NNPC_out"=w147:T27, "dT_Coreset"=w150:dbl)  [unwired: 3 in]
          "dT_Coreset" <- w150
          n33 = for "Coreset Size" {
            N -> [w210]
            tunnel: w188 -> [w218]
            shift-right: [w217] -> w185
            shift-left: w147 -> [w196]
            shift-right: [w189] -> w182
            shift-left: w148 -> [w194]
            tunnel: w181 -> [w231]
            tunnel: w180 -> [w220]
            tunnel: w179 -> [w216]
            tunnel: w177 -> [w211]
            tunnel: [w208] -> w170
            shift-right: [w204] -> w168
            shift-left: w169 -> [w205]
            tunnel: [w203] -> w165 mode=indexing
            tunnel: [w202] -> w164 mode=indexing
            tunnel: w146 -> [w192] mode=indexing
            i -> [w240]
            stop <- w208 stop-if-true
            w221 = TRUE  # Gen. FP Snapshot?
            w229 = FALSE  # Save?
            n34 = call <vilib>:"NNPC_Shrink_MemBank.vi"("Coreset_Size"=w192, "error in (no error)"=w194, "NNPC_in"=w196) -> ("error out"=w193:errorcluster, "NNPC_out"=w195:T27)  [unwired: 7 in]
            n35 = case shown="True" w229 {
              tunnel: w218 -> [_ w279]
              tunnel: w193 -> [w271 w278]
              tunnel: w195 -> [w272 w277]
              tunnel: [w271 w275] -> w232
              tunnel: [w272 w274] -> w230
              tunnel: w211 -> [_ w273]
              frame False {
              }
              frame True {
                n36 = call <vilib>:"NNPC_Save.vi"("Save_Config"=T24 {"Add_TimeStamp_SubFolder"=TRUE, "Append_TimeStamp_to_FileNames"=TRUE} ("Save Config"), "Dst_Folder"=w279, "error in (no error)"=w278, "PreProc_Options_in"=w273, "NNPC_in"=w277) -> ("error out"=w275:errorcluster, "NNPC_out"=w274:T27)  [unwired: 4 in, 1 out]
              }
            }
            n37 = local read "DS Size(Test)"() -> (w227:i32)
            n38 = call-poly <vilib>:"NNPC_Predict.vi"("Dataset"=w231, "Feature_Scorer_Params"="Feature_Scorer_Params", "error in (no error)"=w232, "NNPC_in"=w230) -> ("error out"=w235:errorcluster, "Anomaly_Maps"=w234:sgl[][][], "Pred_Scores"=w236:sgl[], "NNPC_out"=w237:T27, "dT_Predict"=w203:dbl)  [unwired: 3 in]
            "dT_Predict" <- w203
            n39 = Divide(x=w203, y=w227) -> (x/y=→"dT_Inference":dbl)
            n40 = call <vilib>:"NNPC_Eval.vi"("Eval_Config"=T21 {"Extract_Good_Pixels_from_Bad"=FALSE, "# bins"=100} ("Eval Config"), "Dataset"=w231, "error in (no error)"=w235, "Anomaly_Maps"=w234, "Pred_Scores"=w236, "NNPC_in"=w237) -> ("error out"=w209:errorcluster, "Evaluation_Metrics"=w206:T44, "NNPC_out"=w217:T27, "dT_Eval"=w202:dbl)  [unwired: 2 in]
            "dT_Eval" <- w202
            n41 = Unbundle By Name(w206) -> ("Evaluation_Metrics(Image)"=w199:T13, "Evaluation_Metrics(Pixel)"=w198:T13)
            n42 = flat-sequence {
              tunnel: w202 -> [w257]
              tunnel: [w257] -> w207
              tunnel: w198 -> [w256]
              tunnel: w199 -> [w255]
              tunnel: [w263] -> w226
              tunnel: [w262] -> w214
              tunnel: [w261] -> w213
              tunnel: [w260] -> w212
              tunnel: w207 -> [_]
              tunnel: [w259] -> w197
              tunnel: [w258] -> w191
              frame #0 {
                "Evaluation_Metrics(Image)" <- w255
                "Evaluation_Metrics(Pixel)" <- w256
              }
              frame #1 {
                n43 = local read "[LayerID, PatchSize]"() -> (w258:cluster{"Layer_ID":i32, "Patch_Size":i32}[])
                n44 = local read "Feature Extractor"() -> (w259:string)
                n45 = local read "Proj. Dim."() -> (w260:i32)
                n46 = local read "Coreset Size"() -> (w261:sgl)
                n47 = local read "dT_Inference"() -> (w262:dbl)
                n48 = local read "dT_Init"() -> (w266:dbl)
                n49 = local read "dT_Embed"() -> (w265:dbl)
                n50 = local read "dT_Coreset"() -> (w264:dbl)
                n51 = Compound Arithmetic op=ADD(w266, w265, w264) -> (w263:dbl)
              }
            }
            n52 = flat-sequence {
              frame #0 {
                n53 = local read "Image Res."() -> (w254:i32[])
                n54 = local read "Feature_Layers"() -> (w246:T11[])
                n55 = local read "Proj._Dim."() -> (w253:i32[])
                n56 = local read "Coreset_Size"() -> (w252:sgl[])
                n57 = local read "NNFE_Folder_Paths"() -> (w245:path[])
                n58 = Array Size(array=w254) -> (size(s)=w250:i32)
                n59 = Array Size(array=w246) -> (size(s)=w251:i32)
                n60 = Array Size(array=w253) -> (size(s)=w249:i32)
                n61 = Array Size(array=w252) -> (size(s)=w248:i32)
                n62 = Array Size(array=w245) -> (size(s)=w244:i32)
                n63 = Compound Arithmetic op=MULTIPLY(w250, w251, w249, w248, w244) -> (→"Total Iters":i32)
              }
            }
            n64 = Unbundle By Name(w217) -> ("NN.Dims_In"=w223:T3, "Name"=w222:string)
            n65 = Unbundle By Name(w199) -> ("Eval Stats"=w225:T14)
            n66 = Unbundle By Name(w198) -> ("Eval Stats"=w224:T14)
            n67 = Bundle By Name(cluster=T22 {"Name"="", "Feature Extractor"="wrn_50_2_2_bnmerge", "Input3D_Custom_Dims"={"C"=0, "H"=0, "W"=-1}, "Coreset Size"=0, "J-L Proj. Dim."=0, "Train_Time"=0.0, "Inf_Time"=0.0, "Feature_Layers"=[{"Layer_ID"=8, "Patch_Size"=3}, {"Layer_ID"=16, "Patch_Size"=3}], "Eval Stats(Image)"={"Scores(Good)"={"Min"=0.0, "Max"=0.0}, "Scores(Bad)"={"Min"=0.0, "Max"=0.0}, "# of Samples(Good)"=0, "# of Samples(Bad)"=0, "AUROC"=0.0, "F1_Max"=0.0, "Thrshld(F1_Max)"=0.0, "Prec.(F1_Max)"=0.0, "Recall(F1_Max)"=0.0, "FPR(F1_Max)"=0.0, "FNR(F1_Max)"=0.0}, "Eval Stats(Pixel)"={"Scores(Good)"={"Min"=0.0, "Max"=0.0}, "Scores(Bad)"={"Min"=0.0, "Max"=0.0}, "# of Samples(Good)"=0, "# of Samples(Bad)"=0, "AUROC"=0.0, "F1_Max"=0.0, "Thrshld(F1_Max)"=0.0, "Prec.(F1_Max)"=0.0, "Recall(F1_Max)"=0.0, "FPR(F1_Max)"=0.0, "FNR(F1_Max)"=0.0}} ("Model_Info_and_Report"), "Feature_Layers"=w191, "Feature Extractor"=w197, "J-L Proj. Dim."=w212, "Coreset Size"=w213, "Inf_Time"=w214, "Train_Time"=w226, "Input3D_Custom_Dims"=w223, "Name"=w222, "Eval Stats(Image)"=w225, "Eval Stats(Pixel)"=w224) -> (w239:T22)
            n68 = Increment(x=w205) -> (x+1=w204:i32)
            n69 = call <vilib>:"NN_Get_T_dT.vi"("T_in"=w216, "error in (no error)"=w209) -> ("error out"=w201:errorcluster, "dT"=→"Elapsed Time":dbl)  [unwired: 5 in, 1 out]
            n70 = call "Model_Info_and_Report_Data(JSON)(Write).vi"("Dest Folder"=w218, "error in (no error)"=w201, "Model_Info_and_Report"=w239) -> ("error out"=w200:errorcluster, "Generated File Path"=w219:path)  [unwired: 7 in]
            n71 = case shown="True" w221 {
              tunnel: w220 -> [_ w268]
              tunnel: w219 -> [_ w267]
              tunnel: w200 -> [_ w269]
              frame False {
              }
              frame True {
                n72 = control-ref of="Tab Control"() -> (w270:refnum<vi>)
                n73 = call "Generate_FP_Snapshot.vi"("TabControl in"=w270, "directory copy"=w268, "error in"=w269, "Generated File Path"=w267) -> ()  [unwired: 7 in, 1 out]
              }
            }
            n74 = flat-sequence {
              tunnel: [w242] -> w208
              tunnel: w200 -> [w241]
              tunnel: [w241] -> w189
              frame #0 {
                n75 = Or(x=w241, y="Stop") -> (x .or. y?=w242:bool)
              }
            }
            "Coreset Size" <- w240
            "Coreset Size" <- w210
            "Current Iter" <- w205
            "Coreset Size" <- w192
          }
          n76 = call <vilib>:"NNPC_Destroy.vi"("error in"=w182, "NNPC_in"=w185) -> ("error out"=w162:errorcluster)  [unwired: 9 in]
          n77 = Or(x=w162, y=w170) -> (x .or. y?=w163:bool)
          "Proj. Dim." <- w186
          "Proj. Dim." <- w178
          "Proj. Dim." <- w171
        }
        n78 = Or(x=w130, y=w121) -> (x .or. y?=w122:bool)
        "Feature_Layers" <- w134
        "Feature_Layers" <- w131
      }
      n79 = Unbundle By Name(w105) -> ("Dataset_Size"=→"DS Size(Test)":i32)
      n80 = Unbundle By Name(w104) -> ("Dataset_Size"=→"DS Size(Train)":i32)
      n81 = Or(x=w89, y=w80) -> (x .or. y?=w81:bool)
      n82 = call-poly <vilib>:"NN_Dataset_Destroy.vi"("error in (no error)"=w80, "Dataset(In3D_Out3D)"=w105) -> ("error out"=w109:errorcluster)  [unwired: 9 in]
      n83 = call-poly <vilib>:"NN_Dataset_Destroy.vi"("error in (no error)"=w80, "Dataset(In3D_Out3D)"=w104) -> ("error out"=w103:errorcluster)  [unwired: 9 in]
      n84 = Merge Errors(w109, w103) -> (w99:errorcluster)
      "Img Res." <- w118
      "Img. Res." <- w115
      "Img Res." <- w90
    }
    "NNFE" <- w50
    "NNFE" <- w49
  }
  "error out" <- w12
  n85 = Add Array Elements(numeric array=w26) -> (sum=→"dT_DS_Read(Train)":dbl)
  n86 = Add Array Elements(numeric array=w25) -> (sum=→"dT_DS_Read(Test)":dbl)
  n87 = Add Array Elements(numeric array=w24) -> (sum=→"dT_Init":dbl)
  n88 = Add Array Elements(numeric array=w8) -> (sum=→"dT_Embed":dbl)
  n89 = Add Array Elements(numeric array=w23) -> (sum=→"dT_Coreset":dbl)
  n90 = Add Array Elements(numeric array=w22) -> (sum=→"dT_Predict":dbl)
  n91 = Add Array Elements(numeric array=w6) -> (sum=→"dT_Eval":dbl)
